vi "Main Page.vi"(8 "error in (no error)":errorcluster, 11 "Node Ptr":T7 format="%.0x") -> (0 "error out":errorcluster)   [LabVIEW 2020, in "Modbus Master System Explorer.lvlib"]
uses:
  Modbus Master System Explorer.lvlib
  <vilib>/NI VeriStand/Custom Device API/Custom Device Item Ref.ctl
  Shared/Controls/Interface Type.ctl
  Shared/Controls/Parity.ctl
  Shared/Controls/Serial Type.ctl
  Shared/Controls/Flow Control.ctl
  SubVIs/Radix.ctl
  Shared/Write Mode.ctl
  Shared/Constants.vi
  <vilib>/NI VeriStand/Custom Device API/Set Item Property (U16).vi
  <vilib>/NI VeriStand/Custom Device API/Custom Device API.lvlib
  Shared/Modbus Master Shared.lvlib
panel:
  in  "Write Refresh Rate (ms)":i32
  in  "Write Mode":T1
  in  "WebBrowser":refnum<k7>(container)
  in  "Maximum Channels per Read":i32
  in  "Read Refresh Rate (ms)":i32
  in  "Export to Kepware Server":bool
  in  "Name":string
  in  "Master Settings Tabs":enum32{"TCP Master", "Serial Master"}(tab)
  in  "Timeout (ms)":i32
  in  "Address":string
  in  "Port":u16
  in  "Baud Rate":string(combo)
  in  "Radix":T2
  in  "Unit ID":u16
  out "Data Bits":u32=7
  in  "VISA resource name":refnum<visa-resource-name>
  in  "flow control (none)":T3 items=["None", "XON/XOFF", "RTS/CTS", "XON/XOFF & RTS/CTS", "DTR/DSR", "XON/XOFF & DTR/DSR"]
  in  "parity (even)":T4=2 items=["None", "Odd", "Even", "Mark", "Space"]
  in  "serial type":T5
  out "Stop Bits":u32
  in  "Wire Mode":i16(ring)=-1 items=["Unknown"=-1, "RS485/Wire4"=0, "RS485/Wire2-EchoDTR"=1, "RS485/Wire2-CtrlDTR"=2, "RS485/Wire2-Auto"=3, "RS232/DTE"=128, "RS232/DCE"=129, "RS232/AUTO"=130]
  in  "Interface Type":T6
  in  "Header":cluster{"Section Name":string}={"Section Name"="Modbus Master to Slave Settings"}
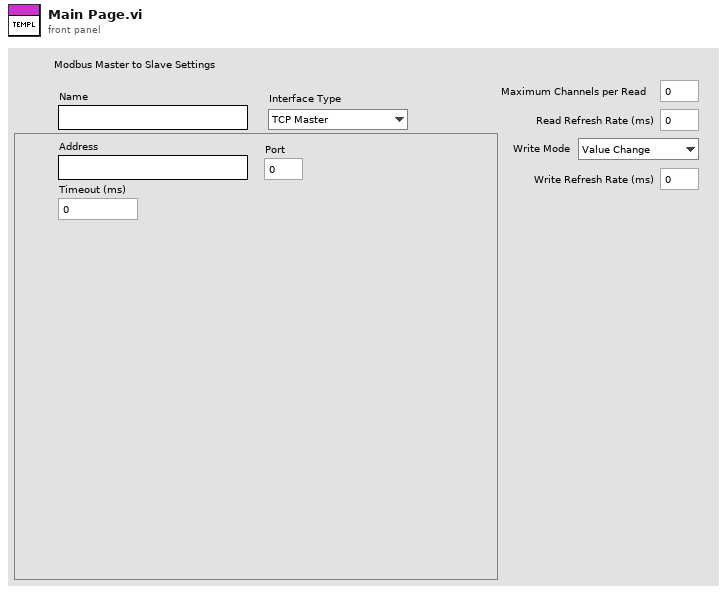
[diagram p1: front panel]
types:
  T1 = typedef "Modbus Master Shared.lvlib/Write Mode.ctl" = enum16{"Value Change", "Interval"}
  T2 = typedef "Modbus Master System Explorer.lvlib/Radix.ctl" = enum32{"Decimal", "Hexidecimal"}
  T3 = typedef "Modbus Master Shared.lvlib/Flow Control.ctl" = u16
  T4 = typedef "Modbus Master Shared.lvlib/Parity.ctl" = u16
  T5 = typedef "Modbus Master Shared.lvlib/Serial Type.ctl" = enum16{"RTU", "ASCII"}
  T6 = typedef "Modbus Master Shared.lvlib/Interface Type.ctl" = enum16{"TCP Master", "Serial Master", "TCP Slave", "Serial Slave"}
  T7 = typedef "Custom Device API.lvlib/Custom Device Item Ref.ctl" = u64
  T8 = enum8{"Enabled", "Disabled", "Disabled and Grayed Out"}
  T9 = typedef "Custom Device API.lvlib/Custom Device Commands.ctl" = enum16{"Default", "Item renamed", "Shutdown", "Dynamic button pressed"}
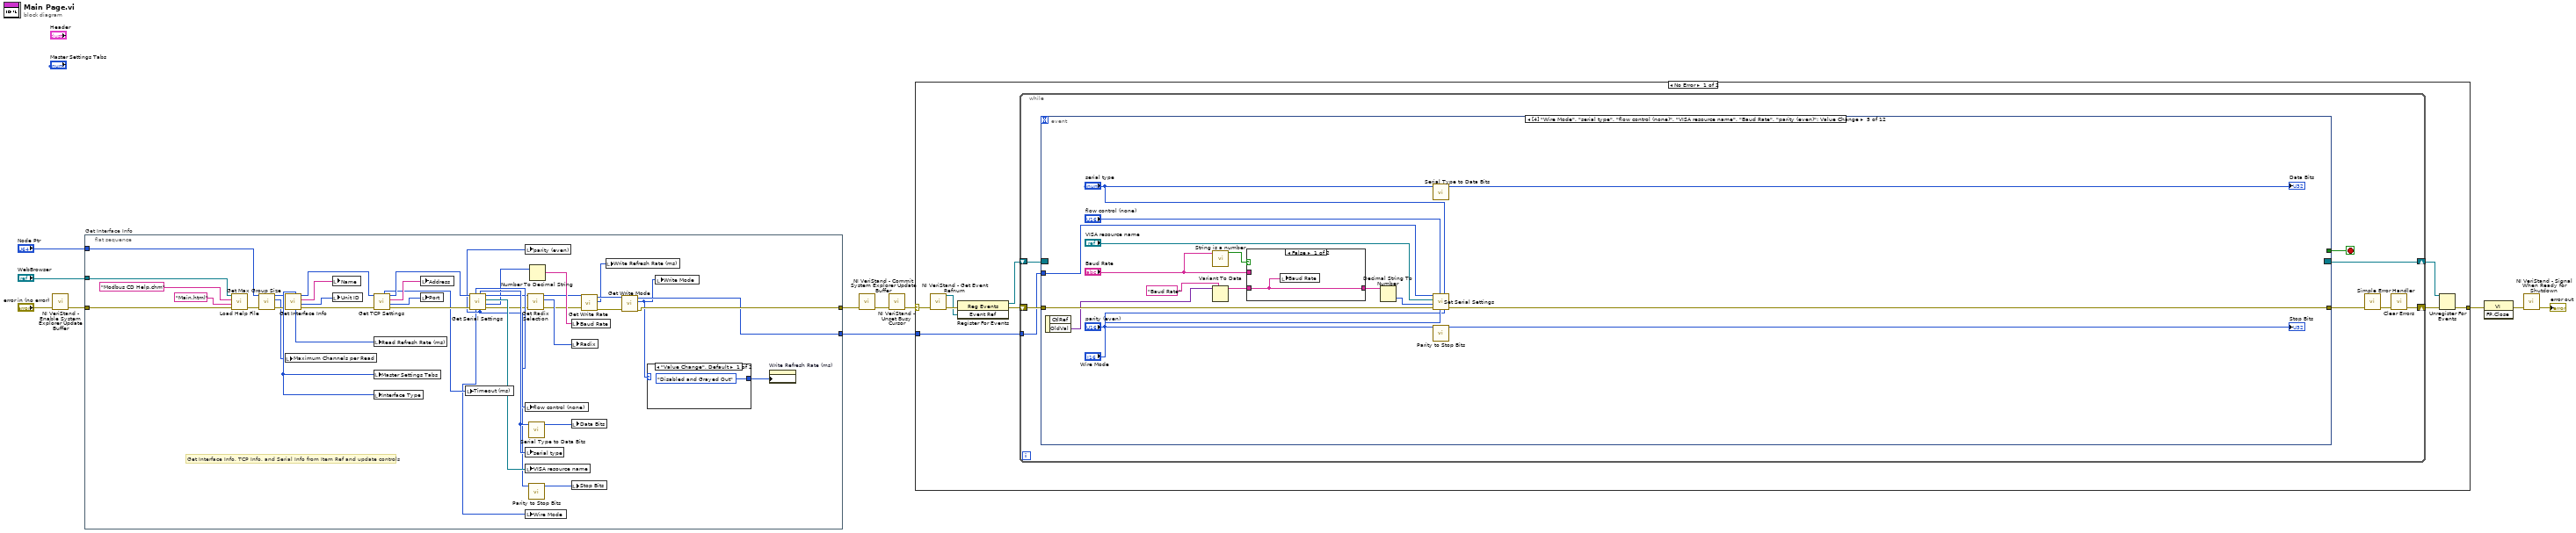
[diagram p0: block diagram]
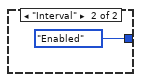
[diagram p2: hidden frame]
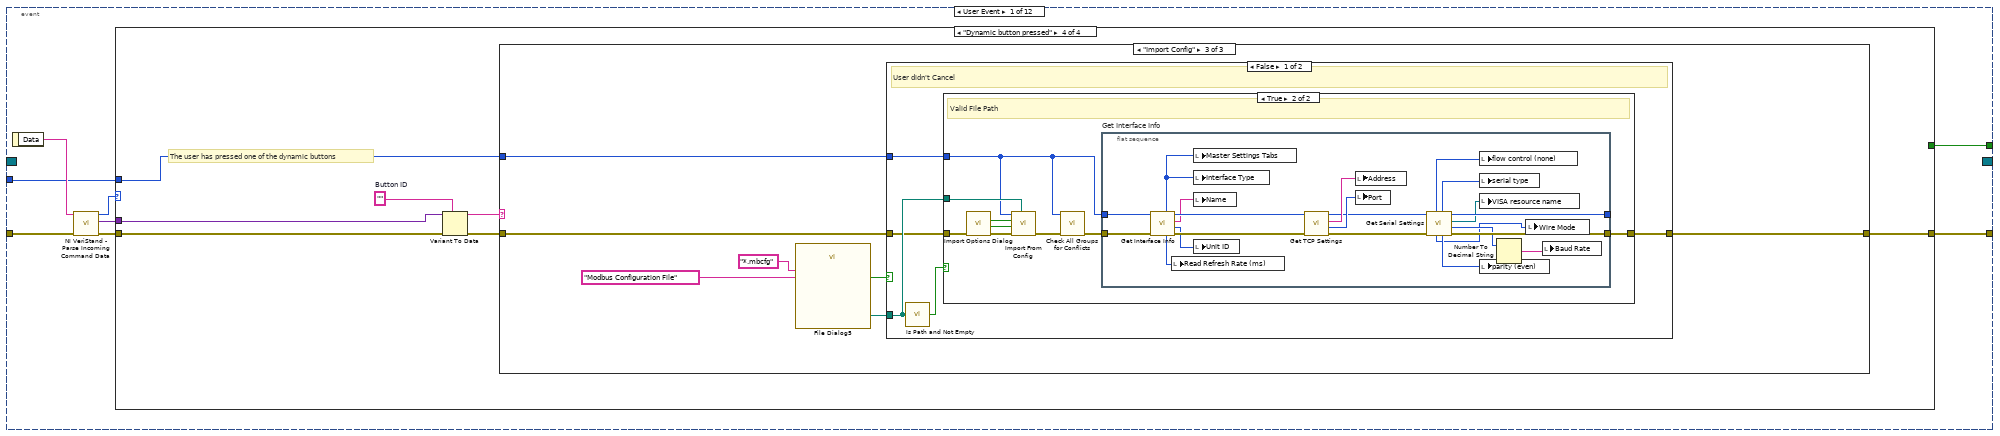
[diagram p3: hidden frame]
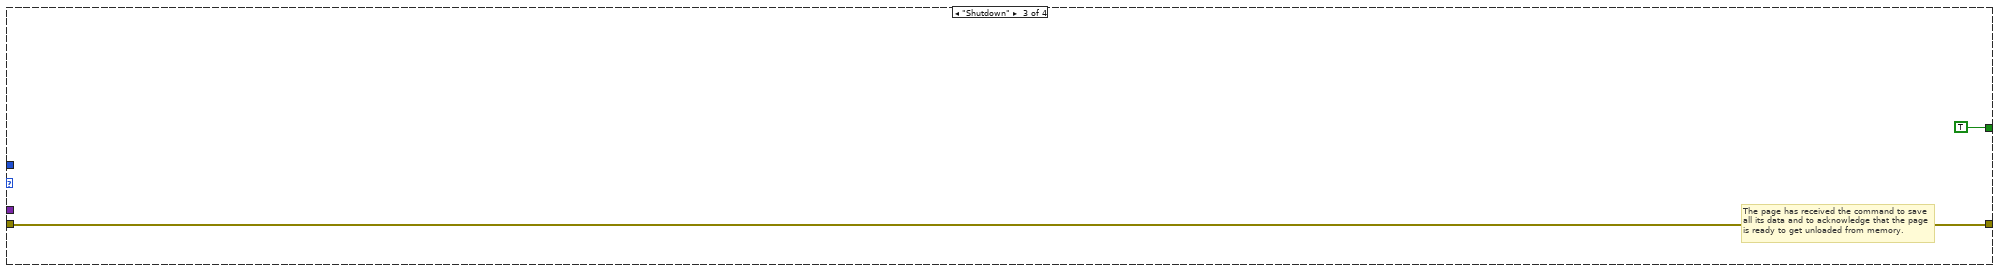
[diagram p6: hidden frame]
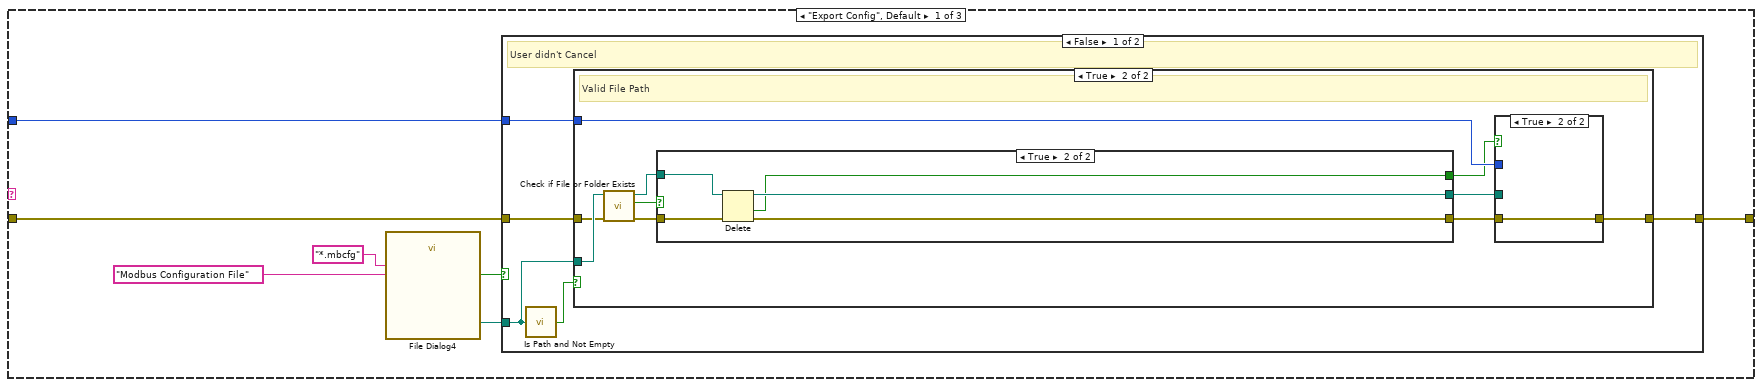
[diagram p7: hidden frame]
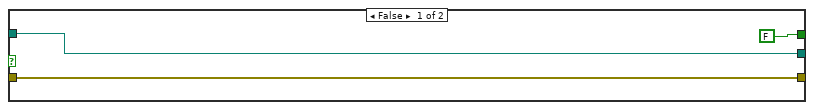
[diagram p9: hidden frame]
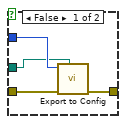
[diagram p10: hidden frame]
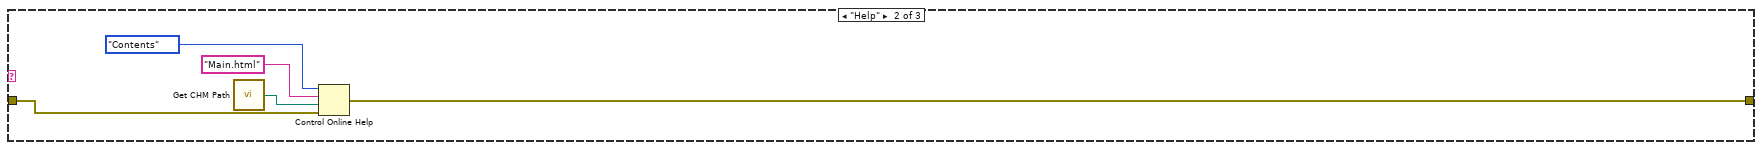
[diagram p12: hidden frame]
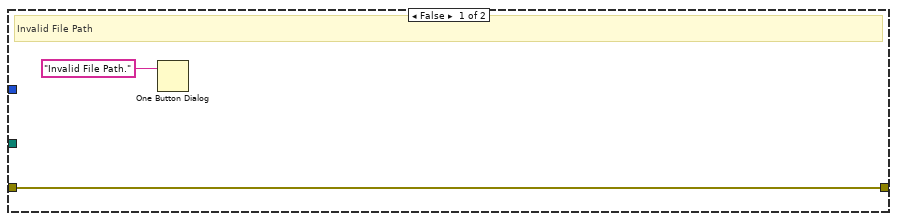
[diagram p13: hidden frame]
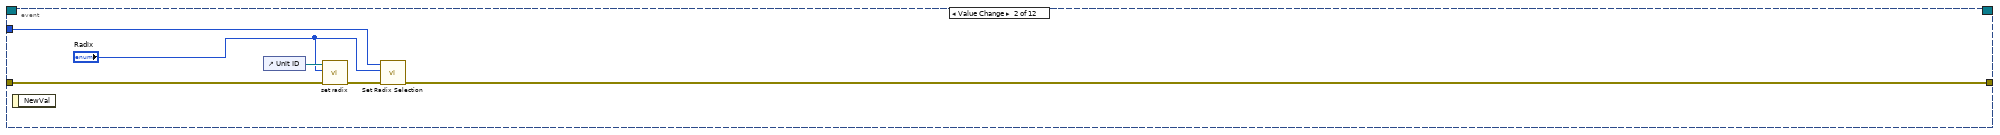
[diagram p15: hidden frame]
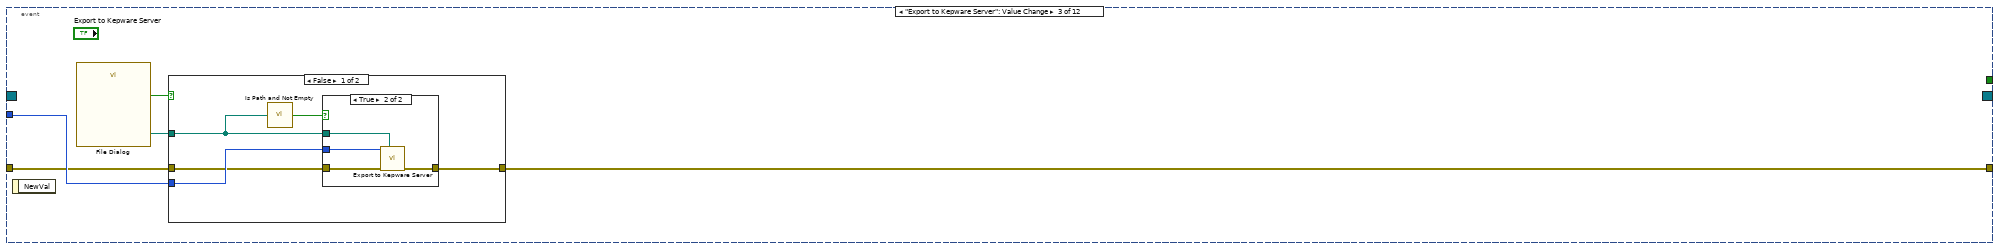
[diagram p16: hidden frame]
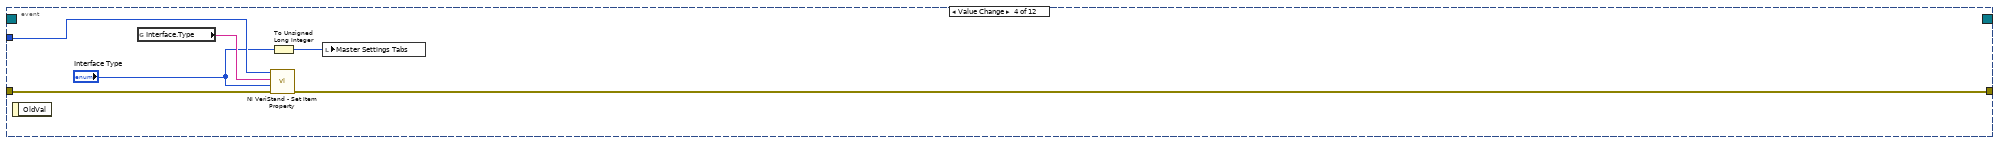
[diagram p19: hidden frame]
diagram:
  n1 = call <vilib>:"NI VeriStand - Enable System Explorer Update Buffer.vi"("error in (no error)"="error in (no error)") -> ("error out"=w1:errorcluster)  [unwired: 10 in]
  n2 = flat-sequence "Get Interface Info" {
    tunnel: w1 -> [w23]
    tunnel: "Node Ptr" -> [w36]
    tunnel: [w18] -> w4
    tunnel: [w15] -> w6
    tunnel: "WebBrowser" -> [w26]
    frame #0 {
      # "Get Interface Info, TCP Info, and Serial Info from Item Ref and update controls"
      n3 = call "Load Help File.vi"("error in (no error)"=w23, "HTML File"="Main.html", "Main CHM File"="Modbus CD Help.chm", "SHDocVw.IWebBrowser2"=w26) -> ("error out"=w22:errorcluster)  [unwired: 7 in]
      n4 = call "Get Max Group Size.vi"("error in (no error)"=w22, "Item Ref in"=w36) -> ("error out"=w34:errorcluster, "Value"=w33:i32, "Item Ref out"=w35:T7)  [unwired: 7 in]
      n5 = local write "Maximum Channels per Read"(w33) -> ()
      n6 = call "Get Interface Info.vi"("error in (no error)"=w34, "Device Item Ref in"=w35) -> ("error out"=w45:errorcluster, "Unit ID"=w42:u16, "Name"=w43:string, "Item Ref out"=w46:T7, "Refresh Rate"=w41:i32, "Interface Type"=w44:T6)  [unwired: 4 in]
      n7 = local write "Name"(w43) -> ()
      n8 = local write "Unit ID"(w42) -> ()
      n9 = call "Get TCP Settings.vi"("error in (no error)"=w45, "Item Ref in"=w46) -> ("error out"=w50:errorcluster, "Port"=w51:u16, "Address"=w52:string, "Item Ref out"=w49:T7, "Timeout"=w32:i32)  [unwired: 5 in]
      n10 = local write "Read Refresh Rate (ms)"(w41) -> ()
      n11 = local write "Master Settings Tabs"(w44) -> ()
      n12 = local write "Interface Type"(w44) -> ()
      n13 = local write "Address"(w52) -> ()
      n14 = local write "Port"(w51) -> ()
      n15 = local write "Timeout (ms)"(w32) -> ()
      n16 = call "Get Serial Settings.vi"("error in (no error)"=w50, "Item Ref in"=w49) -> ("error out"=w31:errorcluster, "baud rate"=w28:u32, "VISA resource name"=w47:refnum<visa-resource-name>, "Item Ref out"=w30:T7, "parity (even)"=w38:T4, "serial type"=w39:T5, "Wire Mode"=w21:i32, "flow control (none)"=w48:T3)  [unwired: 2 in]
      n17 = local write "parity (even)"(w38) -> ()
      n18 = local write "flow control (none)"(w48) -> ()
      n19 = local write "serial type"(w39) -> ()
      n20 = local write "VISA resource name"(w47) -> ()
      n21 = local write "Wire Mode"(w21) -> ()
      n22 = call "Get Radix Selection.vi"("error in (no error)"=w31, "Item Ref in"=w30) -> ("error out"=w20:errorcluster, "Radix"=w29:T2, "Item Ref out"=w17:T7)  [unwired: 7 in]
      n23 = call "Serial Type to Data Bits.vi"("serial type"=w39) -> ("Data Bits"=w40:u32)  [unwired: 10 in]
      n24 = call "Parity to Stop Bits.vi"("parity"=w38) -> ("Stop Bits"=w37:u32)  [unwired: 10 in]
      n25 = Number To Decimal String(number=w28) -> (decimal integer string=w27:string)  [unwired: 1 in]
      n26 = local write "Baud Rate"(w27) -> ()
      n27 = local write "Radix"(w29) -> ()
      n28 = local write "Data Bits"(w40) -> ()
      n29 = local write "Stop Bits"(w37) -> ()
      n30 = call "Get Write Rate.vi"("error in (no error)"=w20, "Item Ref in"=w17) -> ("error out"=w19:errorcluster, "Value"=w14:i32, "Item Ref out"=w16:T7)  [unwired: 7 in]
      n31 = local write "Write Refresh Rate (ms)"(w14) -> ()
      n32 = call "Get Write Mode.vi"("error in (no error)"=w19, "Item Ref in"=w16) -> ("error out"=w18:errorcluster, "Write Mode"=w12:T1, "Item Ref out"=w15:T7)  [unwired: 7 in]
      n33 = case shown="\"Value Change\", Default" w12 {
        tunnel: [T8."Disabled and Grayed Out" ("Disabled") T8."Enabled" ("Disabled")] -> w13
        frame "Value Change", Default {
        }
        frame "Interval" {
        }
      }
      n34 = local write "Write Mode"(w12) -> ()
      n35 = property on="Write Refresh Rate (ms)" class="DigNum (strict)"("DisabledEnum"=w13) -> ()  [unwired: 2 in, 2 out]
    }
  }
  n36 = call <vilib>:"NI VeriStand - Commit System Explorer Update Buffer.vi"("error in (no error)"=w4) -> ("error out"=w3:errorcluster)  [unwired: 10 in]
  n37 = call <vilib>:"NI VeriStand - Unset Busy Cursor.vi"("error in (no error)"=w3) -> ("error out"=w7:errorcluster)  [unwired: 10 out]
  n38 = case shown="No Error" w7 {
    selector: w7 -> [w55 w258]
    tunnel: [w60 w256] -> w11
    tunnel: w6 -> [w56 _]
    frame No Error {
      n39 = call <vilib>:"NI VeriStand - Get Event Refnum.vi"("error in (no error)"=w55) -> ("error out"=w63:errorcluster, "Event Ref"=w59:refnum<user-event>)  [unwired: 9 out]
      n40 = register-events(error in=w63, w59) -> (reference out=w57:refnum<event-registration>, error out=w58:errorcluster)  [unwired: 1 in]
      n41 = while {
        tunnel: w56 -> [w67]
        shift-right: [w64] -> w61
        shift-left: w58 -> [w70]
        shift-right: [w71] -> w62
        shift-left: w57 -> [w69]
        stop <- w68 stop-if-true
        n42 = event shown="[4] \"Wire Mode\", \"serial type\", \"flow control (none)\", \"VISA resource name\", \"Baud Rate\", \"parity (even)\": Value Change" {
          selector: w69 -> [_ _ _ _ _ _ _ _ _ _ _ _]
          dyn-events: [_ _ _ _ _ _ _ _ _ _ _ _] -> w71
          timeout: _ -> [_ _ _ _ _ _ _ _ _ _ _ _]
          tunnel: w70 -> [w79 w181 w185 w203 w220 w225 w229 w233 w239 w244 w248 w254]
          tunnel: [w75 _ _ _ _ _ _ _ _ _ _ _] -> w68
          tunnel: [w74 w179 w184 w200 w218 _ w228 w232 _ _ w247 w253] -> w66
          tunnel: w67 -> [w73 w183 w186 w204 w221 w227 w231 w234 w240 w245 w249 w255]
          event User Event {
            n43 = event-data() -> ("Data"=w78:string)  [unwired: 1 out]
            n44 = call <vilib>:"NI VeriStand - Parse Incoming Command Data.vi"("error in (no error)"=w79, "Incoming data"=w78) -> ("error out"=w77:errorcluster, "Outgoing data"=w72:variant, "Action"=w76:T9)  [unwired: 7 out]
            n45 = case shown="\"Dynamic button pressed\"" w76 {
              tunnel: w77 -> [w80 w81 w82 w90]
              tunnel: [_ _ TRUE _] -> w75
              tunnel: [w80 w81 w82 w84] -> w74
              tunnel: w73 -> [_ _ _ w86]
              tunnel: w72 -> [_ _ _ w89]
              frame "Default", Default {
              }
              frame "Item renamed" {
              }
              frame "Shutdown" {
                # "The page has received the command to save all its data and to acknowledge that the page is ready to get unloaded from memory."
              }
              frame "Dynamic button pressed" {
                w88 = ""  # Button ID
                # "The user has pressed one of the dynamic buttons"
                n46 = Variant To Data(error in=w90, type=w88, Variant=w89) -> (data=w87:string, error out=w85:errorcluster)
                n47 = case shown="\"Import Config\"" w87 {
                  tunnel: w86 -> [w95 _ w137]
                  tunnel: w85 -> [w94 w129 w136]
                  tunnel: [w93 w128 w135] -> w84
                  frame "Export Config", Default {
                    n48 = call "File Dialog4"("pattern (all files)"="*.mbcfg", "pattern label"="Modbus Configuration File") -> ("selected path"=w97:path, "cancelled"=w96:bool)  [unwired: 10 in, 2 out]
                    n49 = case shown="False" w96 {
                      tunnel: w97 -> [w101 _]
                      tunnel: w95 -> [w100 _]
                      tunnel: w94 -> [w99 w127]
                      tunnel: [w98 w127] -> w93
                      frame False {
                        # "User didn't Cancel"
                        n50 = call <vilib>:"Is Path and Not Empty.vi"("path"=w101) -> ("Is Path and Not Empty?"=w102:bool)  [unwired: 4 in]
                        n51 = case shown="True" w102 {
                          tunnel: w101 -> [_ w108]
                          tunnel: w100 -> [_ w112]
                          tunnel: w99 -> [w103 w105]
                          tunnel: [w103 w113] -> w98
                          frame False {
                          }
                          frame True {
                            # "Valid File Path"
                            n52 = call <vilib>:"Check if File or Folder Exists.vi"("error in (no error)"=w105, "path"=w108) -> ("error out"=w104:errorcluster, "file or folder exists?"=w106:bool, "dup path"=w107:path)  [unwired: 7 in]
                            n53 = case shown="True" w106 {
                              tunnel: [w116 w121] -> w111
                              tunnel: [FALSE ("cancelled") w120] -> w110
                              tunnel: w104 -> [w115 w119]
                              tunnel: [w115 w118] -> w109
                              tunnel: w107 -> [w116 w117]
                              frame False {
                              }
                              frame True {
                                n54 = Delete(path (use dialog)=w117, error in=w119) -> (deleted path=w121:path, cancelled=w120:bool, error out=w118:errorcluster)  [unwired: 3 in]
                              }
                            }
                            n55 = case shown="True" w110 {
                              tunnel: w109 -> [w125 w126]
                              tunnel: [w124 w126] -> w113
                              tunnel: w112 -> [w123 _]
                              tunnel: w111 -> [w122 _]
                              frame False {
                                n56 = call "Export to Config.vi"("selected path"=w122, "error in"=w125, "Device Ref in"=w123) -> ("error out"=w124:errorcluster)  [unwired: 8 in]
                              }
                              frame True {
                              }
                            }
                          }
                        }
                      }
                      frame True {
                      }
                    }
                  }
                  frame "Help" {
                    n57 = call "Get CHM Path.vi"() -> ("appended path"=w132:path)
                    n58 = Control Online Help(1:w129, 2:w132, 3:"Main.html" ("String to search for"), 4:enum16{"Contents", "Key", "Close"}."Contents" ("Operation")) -> (0:w128:errorcluster)
                  }
                  frame "Import Config" {
                    n59 = call "File Dialog5"("pattern (all files)"="*.mbcfg", "pattern label"="Modbus Configuration File") -> ("selected path"=w139:path, "cancelled"=w138:bool)  [unwired: 10 in, 2 out]
                    n60 = case shown="False" w138 {
                      tunnel: w139 -> [w143 _]
                      tunnel: w137 -> [w142 _]
                      tunnel: w136 -> [w141 w177]
                      tunnel: [w140 w177] -> w135
                      frame False {
                        # "User didn't Cancel"
                        n61 = call <vilib>:"Is Path and Not Empty.vi"("path"=w143) -> ("Is Path and Not Empty?"=w144:bool)  [unwired: 4 in]
                        n62 = case shown="True" w144 {
                          tunnel: w143 -> [_ w155]
                          tunnel: w142 -> [_ w153]
                          tunnel: w141 -> [w146 w150]
                          tunnel: [w146 w151] -> w140
                          frame False {
                            # "Invalid File Path"
                            n63 = One Button Dialog(message="Invalid File Path.") -> ()  [unwired: 1 in, 1 out]
                          }
                          frame True {
                            # "Valid File Path"
                            n64 = call "Import Options Dialog.vi"("error in (no error)"=w150) -> ("error out"=w149:errorcluster, "Overwrite Existing Channels?"=w147:bool, "Overwrite Device Settings?"=w148:bool)  [unwired: 8 in]
                            n65 = call "Import From Config.vi"("selected path"=w155, "error in"=w149, "Overwrite Existing Channels?"=w147, "Overwrite Device Settings?"=w148, "Device Ref in"=w153) -> ("error out"=w154:errorcluster)  [unwired: 6 in]
                            n66 = call "Check All Groups for Conflicts.vi"("error in (no error)"=w154, "Item Ref in"=w153) -> ("error out"=w152:errorcluster)  [unwired: 9 in]
                            n67 = flat-sequence "Get Interface Info" {
                              tunnel: w152 -> [w159]
                              tunnel: w153 -> [w160]
                              tunnel: [w173] -> w151
                              tunnel: [w171] -> _
                              frame #0 {
                                n68 = call "Get Interface Info.vi"("error in (no error)"=w159, "Device Item Ref in"=w160) -> ("error out"=w165:errorcluster, "Unit ID"=w162:u16, "Name"=w163:string, "Item Ref out"=w166:T7, "Refresh Rate"=w161:i32, "Interface Type"=w164:T6)  [unwired: 4 in]
                                n69 = local write "Read Refresh Rate (ms)"(w161) -> ()
                                n70 = local write "Master Settings Tabs"(w164) -> ()
                                n71 = local write "Interface Type"(w164) -> ()
                                n72 = local write "Name"(w163) -> ()
                                n73 = local write "Unit ID"(w162) -> ()
                                n74 = call "Get TCP Settings.vi"("error in (no error)"=w165, "Item Ref in"=w166) -> ("error out"=w174:errorcluster, "Port"=w175:u16, "Address"=w176:string, "Item Ref out"=w172:T7)  [unwired: 5 in, 1 out]
                                n75 = local write "Address"(w176) -> ()
                                n76 = local write "Port"(w175) -> ()
                                n77 = call "Get Serial Settings.vi"("error in (no error)"=w174, "Item Ref in"=w172) -> ("error out"=w173:errorcluster, "baud rate"=w158:u32, "VISA resource name"=w167:refnum<visa-resource-name>, "Item Ref out"=w171:T7, "parity (even)"=w170:T4, "serial type"=w169:T5, "Wire Mode"=w156:i32, "flow control (none)"=w168:T3)  [unwired: 2 in]
                                n78 = local write "flow control (none)"(w168) -> ()
                                n79 = local write "serial type"(w169) -> ()
                                n80 = local write "VISA resource name"(w167) -> ()
                                n81 = local write "parity (even)"(w170) -> ()
                                n82 = Number To Decimal String(number=w158) -> (decimal integer string=w157:string)  [unwired: 1 in]
                                n83 = local write "Wire Mode"(w156) -> ()
                                n84 = local write "Baud Rate"(w157) -> ()
                              }
                            }
                          }
                        }
                      }
                      frame True {
                        # "User Canecelled, do nothing"
                      }
                    }
                  }
                }
              }
            }
          }
          event Value Change {
            n85 = event-data() -> ()  [unwired: 2 out]
            n86 = control-ref of="Unit ID"() -> (w182:refnum<vi>)
            n87 = call "set radix.vi"("error in (no error)"=w181, "Radix"="Radix", "Digital in"=w182) -> ("error out"=w180:errorcluster)  [unwired: 8 in]
            n88 = call "Set Radix Selection.vi"("error in (no error)"=w180, "Radix"="Radix", "Item Ref in"=w183) -> ("error out"=w179:errorcluster)  [unwired: 7 in, 1 out]
          }
          event "Export to Kepware Server": Value Change {
            n89 = event-data() -> ()  [unwired: 2 out]
            n90 = call "File Dialog"() -> ("selected path"=w188:path, "cancelled"=w187:bool)  [unwired: 12 in, 2 out]
            n91 = case shown="False" w187 {
              tunnel: w188 -> [w192 _]
              tunnel: w186 -> [w191 _]
              tunnel: w185 -> [w190 w199]
              tunnel: [w189 w199] -> w184
              frame False {
                n92 = call <vilib>:"Is Path and Not Empty.vi"("path"=w192) -> ("Is Path and Not Empty?"=w193:bool)  [unwired: 4 in]
                n93 = case shown="True" w193 {
                  tunnel: w192 -> [_ w198]
                  tunnel: w191 -> [_ w197]
                  tunnel: w190 -> [w194 w196]
                  tunnel: [w194 w195] -> w189
                  frame False {
                  }
                  frame True {
                    n94 = call "Export to Kepware Server.vi"("selected path"=w198, "error in"=w196, "Device Ref in"=w197) -> ("error out"=w195:errorcluster)  [unwired: 8 in]
                  }
                }
              }
              frame True {
              }
            }
          }
          event Value Change {
            n95 = event-data() -> ()  [unwired: 2 out]
            n96 = global read "Constants.vi" "Interface.Type"() -> (w205:string)
            n97 = call-poly <vilib>:"NI VeriStand - Set Item Property.vi"("error in (no error)"=w203, "Value"="Interface Type", "Property Name"=w205, "Item Ref in"=w204) -> ("error out"=w200:errorcluster)  [unwired: 5 in, 2 out]
            n98 = To Unsigned Long Integer(number="Interface Type") -> (unsigned 32bit integer=w202:u32)
            n99 = local write "Master Settings Tabs"(w202) -> ()
          }
          event "Wire Mode", "VISA resource name", "Baud Rate": Value Change {
            n100 = event-data() -> ("OldVal"=w208:variant)  [unwired: 2 out]
            n101 = Variant To Data(type="Baud Rate" ("y"), Variant=w208) -> (data=w207:string)  [unwired: 1 in, 1 out]
            n102 = call "String is a number.vi"("Baud Rate"="Baud Rate") -> ("Boolean"=w211:bool)  [unwired: 10 in]
            n103 = case shown="False" w211 {
              tunnel: "Baud Rate" -> [_ w224]
              tunnel: [w223 w224] -> w209
              tunnel: w207 -> [w223 _]
              frame False {
                n104 = local write "Baud Rate"(w223) -> ()
              }
              frame True {
              }
            }
            n105 = Decimal String To Number(string=w209) -> (number=w215:i32)  [unwired: 2 in, 1 out]
            n106 = call "Serial Type to Data Bits.vi"("serial type"="serial type") -> ("Data Bits"=→"Data Bits":u32)  [unwired: 10 in]
            n107 = call "Set Serial Settings.vi"("Wire Mode"="Wire Mode", "serial type"="serial type", "parity (even)"="parity (even)", "flow control (none)"="flow control (none)", "error in (no error)"=w220, "baud rate"=w215, "VISA resource name"="VISA resource name", "Item Ref in"=w221) -> ("error out"=w218:errorcluster)  [unwired: 2 in, 1 out]
            n108 = call "Parity to Stop Bits.vi"("parity"="parity (even)") -> ("Stop Bits"=→"Stop Bits":u32)  [unwired: 10 in]
          }
          event "Maximum Channels per Read": Value Change {
            n109 = event-data() -> ()  [unwired: 7 out]
            n110 = call "Set Max Group Size.vi"("error in (no error)"=w225, "Value"="Maximum Channels per Read", "Item Ref in"=w227) -> ()  [unwired: 7 in, 2 out]
          }
          event "Name": Value Change {
            n111 = event-data() -> ()  [unwired: 4 out]
            n112 = call "update name.vi"("error in (no error)"=w229, "Desired Alias"="Name", "Parent Ref in"=w231) -> ("error out"=w228:errorcluster)  [unwired: 7 in, 1 out]
          }
          event "Unit ID": Value Change {
            n113 = event-data() -> ()  [unwired: 2 out]
            n114 = global read "Constants.vi" "Interface.UnitID"() -> (w236:string)
            n115 = call-poly <vilib>:"NI VeriStand - Set Item Property.vi"("error in (no error)"=w233, "Value"="Unit ID", "Property Name"=w236, "Item Ref in"=w234) -> ("error out"=w232:errorcluster)  [unwired: 5 in, 2 out]
          }
          event Value Change {
            n116 = event-data() -> ()  [unwired: 7 out]
            n117 = call "Set Write Mode.vi"("error in (no error)"=w239, "Write Mode"="Write Mode", "Item Ref in"=w240) -> ()  [unwired: 7 in, 2 out]
            n118 = case shown="\"Value Change\", Default" "Write Mode" {
              tunnel: [T8."Disabled and Grayed Out" ("Disabled") T8."Enabled" ("Disabled")] -> w237
              frame "Value Change", Default {
              }
              frame "Interval" {
              }
            }
            n119 = property on="Write Refresh Rate (ms)" class="DigNum (strict)"("DisabledEnum"=w237) -> ()  [unwired: 2 in, 2 out]
          }
          event "Write Refresh Rate (ms)": Value Change {
            n120 = event-data() -> ()  [unwired: 7 out]
            n121 = call "Set Write Rate.vi"("error in (no error)"=w244, "Value"="Write Refresh Rate (ms)", "Item Ref in"=w245) -> ()  [unwired: 7 in, 2 out]
          }
          event "Read Refresh Rate (ms)": Value Change {
            n122 = event-data() -> ()  [unwired: 5 out]
            n123 = call "Set Refresh Rate.vi"("error in (no error)"=w248, "Value"="Read Refresh Rate (ms)", "Item Ref in"=w249) -> ("error out"=w247:errorcluster)  [unwired: 7 in, 1 out]
          }
          event "Address", "Port", "Timeout (ms)": Value Change {
            n124 = event-data() -> ()  [unwired: 4 out]
            n125 = call "Set TCP Settings.vi"("Timeout"="Timeout (ms)", "error in (no error)"=w254, "Port"="Port", "Address"="Address", "Item Ref in"=w255) -> ("error out"=w253:errorcluster)  [unwired: 5 in, 1 out]
          }
        }
        n126 = call <vilib>:"Simple Error Handler.vi"("error in (no error)"=w66) -> ("error out"=w65:errorcluster)  [unwired: 1 in, 7 out]
        n127 = call <vilib>:"Clear Errors.vi"("error in (no error)"=w65) -> ("error out"=w64:errorcluster)  [unwired: 1 in, 5 out]
      }
      n128 = Unregister For Events(event registration refnum=w62, error in=w61) -> (error out=w60:errorcluster)
    }
    frame Error {
      n129 = call <vilib>:"Simple Error Handler.vi"("error in (no error)"=w258) -> ("error out"=w257:errorcluster)  [unwired: 1 in, 7 out]
      n130 = call <vilib>:"Clear Errors.vi"("error in (no error)"=w257) -> ("error out"=w256:errorcluster)  [unwired: 1 in, 5 out]
    }
  }
  n131 = invoke class="VI" method="FP.Close"(error in=w11) -> (error out=w10:errorcluster)  [unwired: 2 in, 2 out]
  n132 = call <vilib>:"NI VeriStand - Signal When Ready for Shutdown.vi"("error in (no error)"=w10) -> ("error out"=→"error out":errorcluster)  [unwired: 10 out]
